vi "zad1.vi"() -> ()   [LabVIEW 2017]
panel:
  in  "Stan 6":bool
  in  "Stan 4":bool
  in  "Stan 5":bool
  in  "Stan 3":bool
  in  "Stan 2":bool
  in  "Stan 7":bool
  in  "Stan 1":bool
  in  "Start":bool
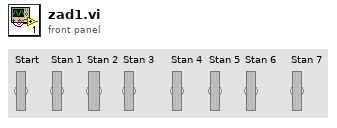
[diagram p1: front panel]
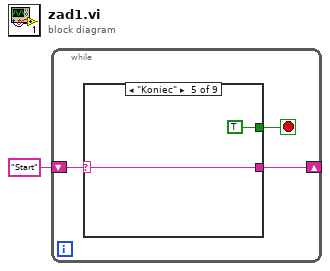
[diagram p0: block diagram]
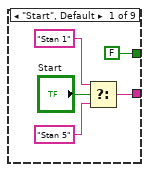
[diagram p2: hidden frame]
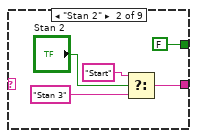
[diagram p3: hidden frame]
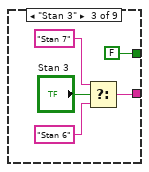
[diagram p4: hidden frame]
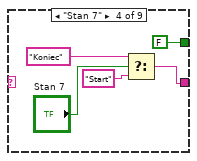
[diagram p5: hidden frame]
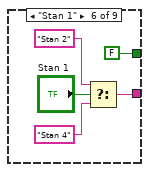
[diagram p6: hidden frame]
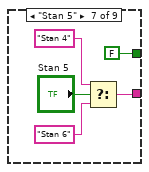
[diagram p7: hidden frame]
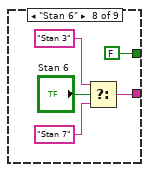
[diagram p8: hidden frame]
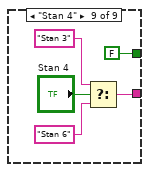
[diagram p9: hidden frame]
diagram:
  n1 = while {
    shift-right: [w3] -> _
    shift-left: "Start" -> [w4]
    stop <- w2 stop-if-true
    n2 = case shown="\"Koniec\"" w4 {
      selector: w4 -> [_ _ _ _ w25 _ _ _ _]
      tunnel: [w6 w11 w17 w21 w25 w28 w33 w37 w42] -> w3
      tunnel: [FALSE FALSE FALSE FALSE TRUE FALSE FALSE FALSE FALSE] -> w2
      frame "Start", Default {
        n3 = Select(t="Stan 1", s="Start", f="Stan 5") -> (s? t:f=w6:string)
      }
      frame "Stan 2" {
        n4 = Select(t="Start", s="Stan 2", f="Stan 3") -> (s? t:f=w11:string)
      }
      frame "Stan 3" {
        n5 = Select(t="Stan 7", s="Stan 3", f="Stan 6") -> (s? t:f=w17:string)
      }
      frame "Stan 7" {
        n6 = Select(t="Koniec", s="Stan 7", f="Start") -> (s? t:f=w21:string)
      }
      frame "Koniec" {
      }
      frame "Stan 1" {
        n7 = Select(t="Stan 2", s="Stan 1", f="Stan 4") -> (s? t:f=w28:string)
      }
      frame "Stan 5" {
        n8 = Select(t="Stan 4", s="Stan 5", f="Stan 6") -> (s? t:f=w33:string)
      }
      frame "Stan 6" {
        n9 = Select(t="Stan 3", s="Stan 6", f="Stan 7") -> (s? t:f=w37:string)
      }
      frame "Stan 4" {
        n10 = Select(t="Stan 3", s="Stan 4", f="Stan 6") -> (s? t:f=w42:string)
      }
    }
  }
